vi "socket_monitor.vi"() -> ()   [LabVIEW 2019]
uses:
  vi.lib/addons/zeromq/monitor_event.ctl
  vi.lib/addons/zeromq/socket_type.ctl
  vi.lib/addons/zeromq/zmq_context.lvclass
  vi.lib/addons/zeromq/zeromq.lvlib
  vi.lib/addons/zeromq/zmq_socket.lvclass
panel:
  out "Events":T2(array[cluster]) {"time" format="%<%X>T"}
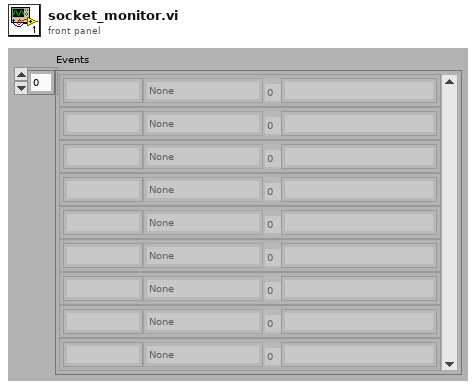
[diagram p1: front panel]
types:
  T1 = typedef "zeromq.lvlib/monitor_event.ctl" = enum8{"None", "Connected", "Connect Delayed", "Connect Retry", "Listening", "Bind Failed", "Accepted", "Accept Failed", "Closed", "Close Failed", "Disconnected"}
  T2 = cluster{"time":timestamp, "event":T1, "addr":string}[]
  T3 = cluster{"seconds since 1Jan1904":timestamp, "event":T1, "addr":string}[]
  T4 = typedef "zeromq.lvlib/socket_type.ctl" = enum8{"ZMQ_PAIR", "ZMQ_PUB", "ZMQ_SUB", "ZMQ_REQ", "ZMQ_REP", "ZMQ_DEALER", "ZMQ_ROUTER", "ZMQ_PULL", "ZMQ_PUSH", "ZMQ_XPUB", "ZMQ_XSUB"}
  T5 = cluster{"seconds since 1Jan1904":timestamp, "event":T1, "addr":string}
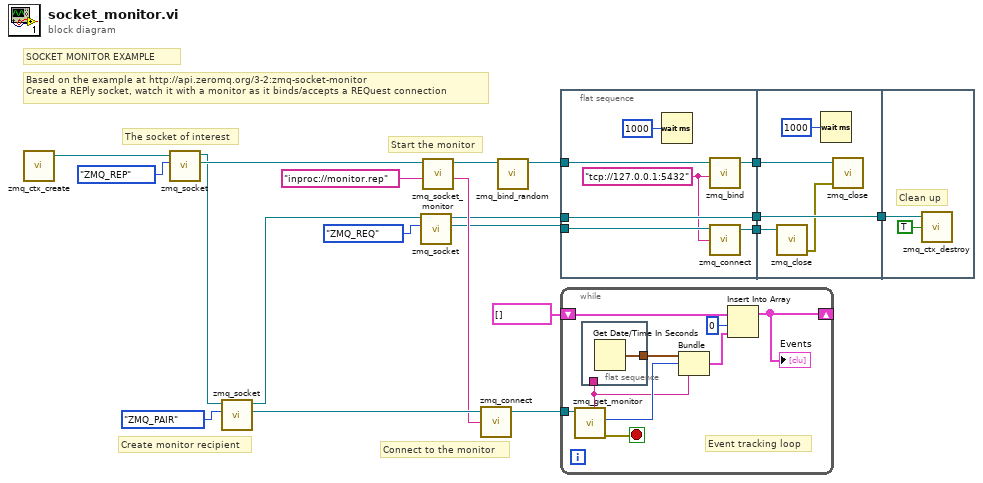
[diagram p0: block diagram]
diagram:
  # "Create monitor recipient"
  # "SOCKET MONITOR EXAMPLE"
  # "Connect to the monitor"
  # "Start the monitor"
  # "The socket of interest"
  # "Based on the example at http://api.zeromq.org/3-2:zmq-socket-monitor\nCreate a REPly socket, watch it with a monitor as it binds/accepts a REQuest connection"
  n1 = call "zmq_ctx_create.vi"() -> ("context out"=w19:refnum<class "zmq_context.lvclass">)  [unwired: 4 in, 1 out]
  n2 = call "zmq_socket.vi"("socket type"=socket_type."ZMQ_REP", "context in"=w19) -> ("socket out"=w18:refnum<class "zmq_socket.lvclass">, "context out"=w12:refnum<class "zmq_context.lvclass">)  [unwired: 3 in, 1 out]
  n3 = call "zmq_socket.vi"("socket type"=socket_type."ZMQ_PAIR", "context in"=w12) -> ("socket out"=w15:refnum<class "zmq_socket.lvclass">, "context out"=w8:refnum<class "zmq_context.lvclass">)  [unwired: 3 in, 1 out]
  n4 = call "zmq_socket.vi"("socket type"=socket_type."ZMQ_REQ", "context in"=w8) -> ("socket out"=w6:refnum<class "zmq_socket.lvclass">, "context out"=w7:refnum<class "zmq_context.lvclass">)  [unwired: 3 in, 1 out]
  n5 = call "zmq_socket_monitor.vi"("endpoint in"="inproc://monitor.rep", "socket in"=w18) -> ("endpoint out"=w14:string, "socket out"=w2:refnum<class "zmq_socket.lvclass">)  [unwired: 2 in, 2 out]
  n6 = call "zmq_connect.vi"("endpoint"=w14, "socket in"=w15) -> ("socket out"=w13:refnum<class "zmq_socket.lvclass">)  [unwired: 2 in, 1 out]
  n7 = call "zmq_bind_random.vi"("socket in"=w2) -> ("socket out"=w1:refnum<class "zmq_socket.lvclass">)  [unwired: 3 in, 3 out]
  n8 = flat-sequence {
    tunnel: w1 -> [w27]
    tunnel: [w26] -> w11
    tunnel: [w24] -> w9
    tunnel: w7 -> [w24]
    tunnel: w6 -> [w23]
    tunnel: [w21] -> w5
    tunnel: w11 -> [w32]
    tunnel: [w30] -> w10
    tunnel: w9 -> [w30]
    tunnel: w5 -> [w29]
    tunnel: w10 -> [w33]
    frame #0 {
      w22 = "tcp://127.0.0.1:5432" ("endpoint")
      n9 = Wait (ms)(milliseconds to wait=u32 1000) -> ()  [unwired: 1 out]
      n10 = call "zmq_bind.vi"("endpoint"=w22, "socket in"=w27) -> ("socket out"=w26:refnum<class "zmq_socket.lvclass">)  [unwired: 2 in, 1 out]
      n11 = call "zmq_connect.vi"("endpoint"=w22, "socket in"=w23) -> ("socket out"=w21:refnum<class "zmq_socket.lvclass">)  [unwired: 2 in, 1 out]
    }
    frame #1 {
      n12 = call "zmq_close.vi"("socket"=w29) -> ("error out"=w28:errorcluster)  [unwired: 4 in]
      n13 = Wait (ms)(milliseconds to wait=u32 1000) -> ()  [unwired: 1 out]
      n14 = call "zmq_close.vi"("error in"=w28, "socket"=w32) -> ()  [unwired: 3 in, 1 out]
    }
    frame #2 {
      # "Clean up"
      n15 = call "zmq_ctx_destroy.vi"("reap? (F)"=TRUE, "context in"=w33) -> ()  [unwired: 3 in, 1 out]
    }
  }
  n16 = while {
    tunnel: w13 -> [w43]
    shift-right: [w36] -> _
    shift-left: T3 [] -> [w37]
    stop <- w42 stop-if-true
    # "Event tracking loop"
    n17 = call "zmq_get_monitor.vi"("monitor in"=w43) -> ("error out"=w42:errorcluster, "event"=w40:T1, "addr"=w39:string)  [unwired: 4 in, 2 out]
    n18 = flat-sequence {
      tunnel: w39 -> [_]
      tunnel: [w44] -> w41
      frame #0 {
        n19 = Get Date/Time In Seconds() -> (seconds since 1Jan1904=w44:timestamp)
      }
    }
    n20 = Bundle("seconds since 1Jan1904"=w41, "event"=w40, "addr"=w39) -> (w38:T5)  [unwired: 1 in]
    n21 = Insert Into Array(array=w37, index=0, new element=w38) -> (w36:T3)
    "Events" <- w36
  }
